vi "Sample_sensor_read.vi"() -> ()   [LabVIEW 2013]
uses:
  <vilib>/Instr/_visa.llb/VISA Configure Serial Port (Instr).vi
panel:
  out "Serial Settings:Number of Bytes at Serial Port":u32
  out "read buffer":string
  out "return count":u32
  out "error out":errorcluster
  in  "write buffer":string="raw_all\\n"
  in  "flow control (0:none)":u16(ring) items=["None", "XON/XOFF", "RTS/CTS", "XON/XOFF & RTS/CTS", "DTR/DSR", "XON/XOFF & DTR/DSR"]
  in  "stop bits (10: 1 bit)":u16(ring)=10 items=["1.0"=10, "1.5"=15, "2.0"=20]
  in  "timeout (10sec)":u32=10000
  in  "error in (no error)":errorcluster
  in  "parity (0:none)":enum16{"None", "Odd", "Even", "Mark", "Space"}(ring)
  in  "data bits (8)":u16=8 min=5 max=8 step=1
  in  "baud rate (9600)":u32=115200
  in  "Port":refnum<visa-resource-name>="COM6"
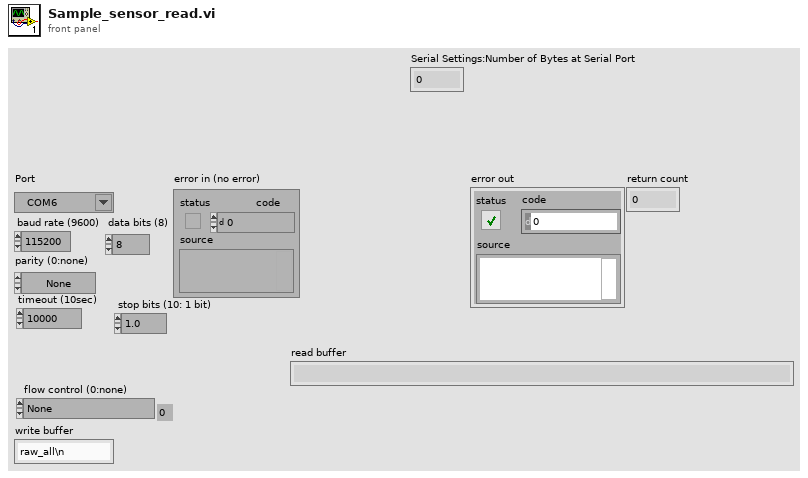
[diagram p1: front panel]
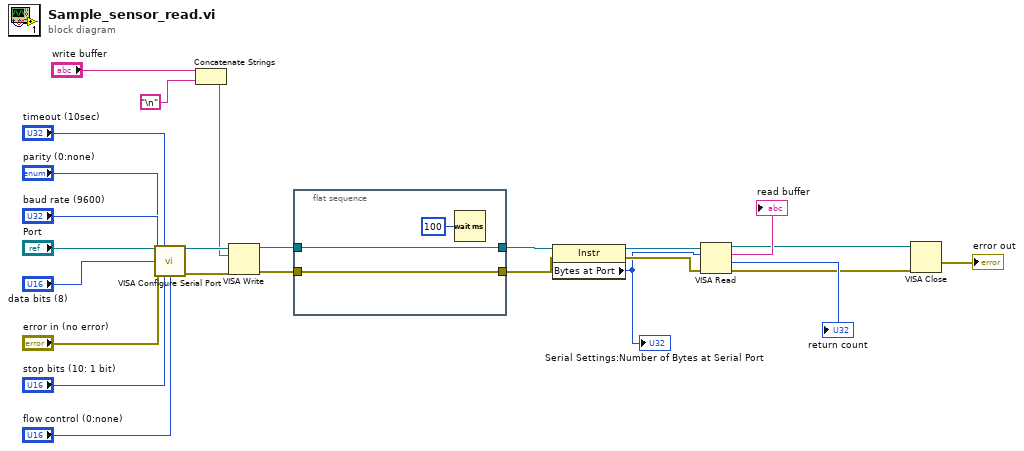
[diagram p0: block diagram]
diagram:
  n1 = call-poly "VISA Configure Serial Port"("VISA resource name"="Port", "timeout (10sec)"="timeout (10sec)", "baud rate (9600)"="baud rate (9600)", "data bits (8)"="data bits (8)", "parity (0:none)"="parity (0:none)", "error in (no error)"="error in (no error)", "stop bits (10: 1 bit)"="stop bits (10: 1 bit)", "flow control (0:none)"="flow control (0:none)") -> ("VISA resource name out"=w17:refnum<visa-resource-name>, "error out"=w16:errorcluster)  [unwired: 6 in]
  n2 = Concatenate Strings("write buffer", "\n") -> (w1:string)
  n3 = VISA Write(VISA resource name=w17, write buffer=w1, error in (no error)=w16) -> (VISA resource name out=w14:refnum<visa-resource-name>, error out=w15:errorcluster)  [unwired: 1 out]
  n4 = flat-sequence {
    tunnel: w15 -> [w27]
    tunnel: [w27] -> w12
    tunnel: w14 -> [w26]
    tunnel: [w26] -> w13
    frame #0 {
      n5 = Wait (ms)(milliseconds to wait=u32 100) -> ()  [unwired: 1 out]
    }
  }
  n6 = property class="Instr"(reference=w13, error in=w12) -> (reference out=w10:refnum<visa-resource-name>, error out=w11:errorcluster, "Bytes at Port"=w4:u32)
  "Serial Settings:Number of Bytes at Serial Port" <- w4
  n7 = VISA Read(VISA resource name=w10, byte count=w4, error in (no error)=w11) -> (VISA resource name out=w5:refnum<visa-resource-name>, read buffer=→"read buffer":string, return count=→"return count":u32, error out=w7:errorcluster)
  n8 = VISA Close(VISA resource name=w5, error in (no error)=w7) -> (error out=→"error out":errorcluster)
